vi "LVUT_MainSequence(Simple Example_Station1).vi"(8 "error in (no error)":errorcluster) -> (0 "error out":errorcluster)   [LabVIEW 2019, in "Simple Example(Station1).lvlib"]
uses:
  Simple Example(Station1).lvlib
  Read Instrument Parameter(Scanner).vi
  Unit Test Engine Tools.lvlib
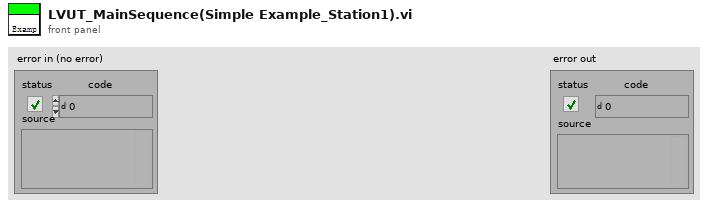
[diagram p1: front panel]
types:
  T1 = enum16{"Station 1", "Station 2", "Station 3", "Station 4"}
  T2 = cluster{"Scanner 1":cluster{"SerialPort":string, "Baud rate":i32, "Address":string, "ID":i32, "Port":i32, "Instrument model":string}, "Scanner 2":cluster{"SerialPort":string, "Baud rate":i32, "Address":string, "ID":i32, "Port":i32, "Instrument model":string}, "Scanner 3":cluster{"SerialPort":string, "Baud rate":i32, "Address":string, "ID":i32, "Port":i32, "Instrument model":string}, "Scanner 4":cluster{"SerialPort":string, "Baud rate":i32, "Address":string, "ID":i32, "Port":i32, "Instrument model":string}}
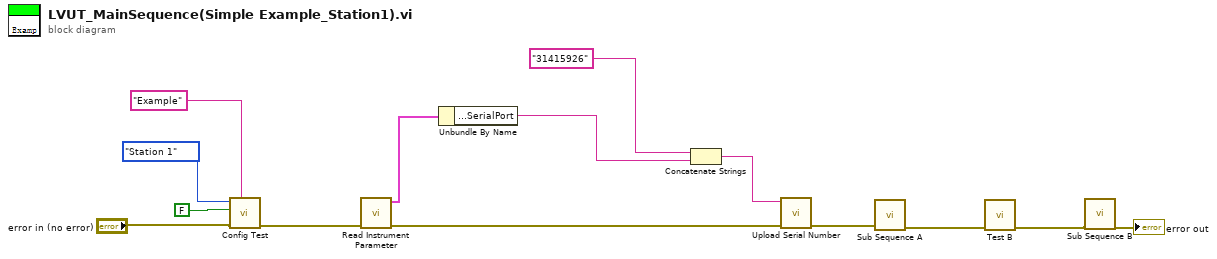
[diagram p0: block diagram]
diagram:
  n1 = call "Config Test.vi"("LimitFileName"="Example", "Error In"="error in (no error)", "Debug"=FALSE, "Station"=T1."Station 1") -> ("Error Out"=w6:errorcluster)  [unwired: 7 in]
  n2 = call-poly "Read Instrument Parameter.vi"("error in (no error)"=w6) -> ("error out"=w5:errorcluster, "Scanner"=w4:T2)  [unwired: 9 in]
  n3 = Unbundle By Name(w4) -> ("Scanner 1.SerialPort"=w2:string)
  n4 = Concatenate Strings("31415926" ("SerialNumber"), w2) -> (w1:string)
  n5 = call "Upload Serial Number.vi"("error in (no error)"=w5, "SerialNumber"=w1) -> ("error out"=w8:errorcluster)  [unwired: 9 in]
  n6 = call "Sub Sequence A.vi"("error in (no error)"=w8) -> ("error out"=w12:errorcluster)  [unwired: 10 in]
  n7 = call "Test B.vi"("error in (no error)"=w12) -> ("error out"=w13:errorcluster)  [unwired: 10 in]
  n8 = call "Sub Sequence B.vi"("error in (no error)"=w13) -> ("error out"=→"error out":errorcluster)  [unwired: 10 in]
